vi "Waveform-Processing-Custom-Device.Async.vi"(10 "Parameters":variant, 11 "Process":refnum<class "Process.lvclass">) -> ()   [LabVIEW 2017, in "Waveform-Processing-Custom-Device Engine.lvlib"]
uses:
  Waveform-Processing-Custom-Device Engine.lvlib
  <vilib>/NI/NIVS Inline Async API/_VS Inline Async API/Process/Process.lvclass
  Shared/CompiledSettings.ctl
  <vilib>/NI Veristand/Custom Device API/Block Data Reference.ctl
  <vilib>/NI Veristand/Custom Device API/Data Reference.ctl
  <vilib>/NI Veristand/Custom Device API/Waveform Data Reference.ctl
  <vilib>/NI/NIVS Inline Async API/_VS Inline Async API/Process/Process.lvclass/Process.ctl
  <vilib>/NI/NIVS Inline Async API/_VS Inline Async API/Process/Data Member Access/Read Data Access.vi
  <vilib>/NI/NIVS Inline Async API/_VS Inline Async API/Error Handling Process/SubVIs/Error.ConvertArray.vi
  <vilib>/NI/NIVS Inline Async API/_Data Access Engine/Data Access Engine/Data Access Engine.lvclass
  Shared/Running Average/Running Average.lvlib
  Shared/Single Point/SinglePoint.lvlib
  <vilib>/NI Veristand/Custom Device API/Custom Device API.lvlib
  Shared/Waveform-Processing-Custom-Device Shared.lvlib
  Shared/Min Single Point/Min_SP.lvlib
  Shared/Max Single Point/Max_SP.lvlib
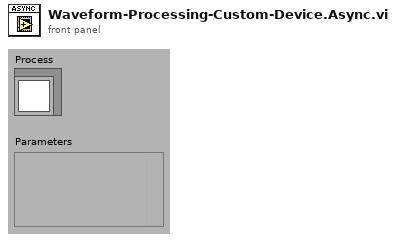
[diagram p1: front panel]
types:
  T1 = typedef "Waveform-Processing-Custom-Device Shared.lvlib/CompiledSettings.ctl" = cluster{"Name":string, "Buffer Length (samples)":u32, "Enable Array":bool[], "Parameter Block Data Refs":T2[], "Source Wfm Data Refs":T4[], "Result Wfm Data Refs":T4[], "Result Ch Data Refs":T3[], "Task Rate (Hz)":dbl}
  T2 = typedef "Custom Device API.lvlib/Block Data Reference.ctl" = cluster{"Data Reference":T3, "Offset":u64, "Length":u64}
  T3 = typedef "Custom Device API.lvlib/Data Reference.ctl" = i32
  T4 = typedef "Custom Device API.lvlib/Waveform Data Reference.ctl" = i32
  T5 = typedef "Waveform-Processing-Custom-Device Engine.lvlib/AsyncStateVariables.ctl" = cluster{"Source Wfm Session Refs":refnum<class "Single Waveform Read (DBL).lvclass">[], "Result Wfm Session Refs":refnum<class "Single Waveform Write (DBL).lvclass">[], "Result Wfm Data":dbl[][], "Source Wfm Data Refs":T4[], "Result Wfm Data Refs":T4[], "Global Buffer Length (samples)":dbl, "Parameter Array":dbl[], "Tag Results":dbl[], "Enable Array":bool[], "Task Rate":dbl, "Data FIFO Refs":T6}
  T6 = typedef "Waveform-Processing-Custom-Device Engine.lvlib/New Async FIFOs.ctl" = cluster{"Single Point Result":T7, "Running Average Result":T7, "Min Single Point Result":T7, "Max Single Point Result ":T7}
  T7 = typedef "Data Access Engine.lvlib/Data Access Engine.lvclass/Write.DVR.ctl" = refnum<data-value>
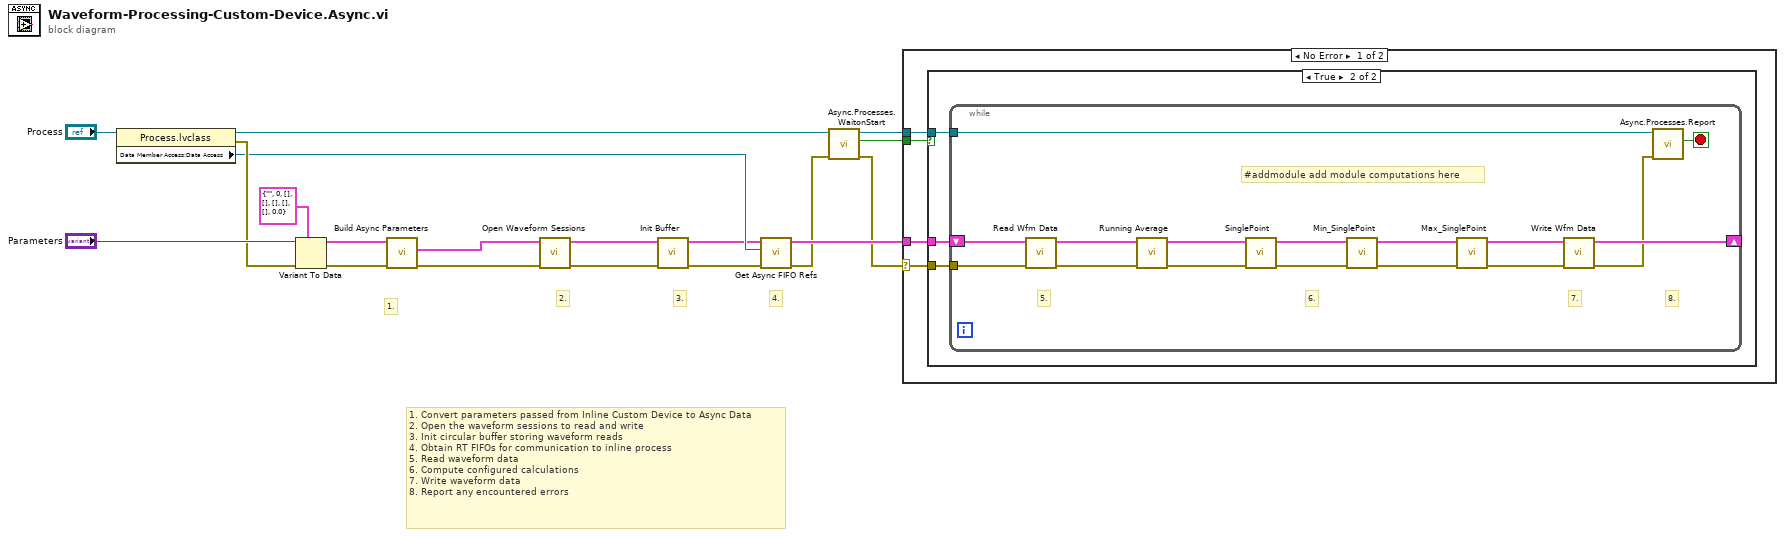
[diagram p0: block diagram]
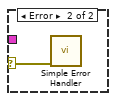
[diagram p3: hidden frame]
diagram:
  # "4."
  # "3."
  # "2."
  # "1."
  # "1. Convert parameters passed from Inline Custom Device to Async Data\n2. Open the waveform sessions to read and write\n3. Init circular buffer storing waveform reads\n4. Obtain RT FIFOs for communication to inline process\n5. Read waveform data\n6. Compute configured calculations\n7. Write waveform data\n8. Report any encountered errors"
  n1 = property class="Process.lvclass"(reference="Process") -> (reference out=w16:refnum<class "Process.lvclass">, error out=w14:errorcluster, "Data Member Access:Data Access"=w12:refnum<class "Data Access Engine.lvclass">)  [unwired: 1 in]
  n2 = Variant To Data(error in=w14, type=T1 {"Name"="", "Buffer Length (samples)"=0, "Enable Array"=[], "Parameter Block Data Refs"=[], "Source Wfm Data Refs"=[], "Result Wfm Data Refs"=[], "Result Ch Data Refs"=[], "Task Rate (Hz)"=0.0} ("CompiledSettings"), Variant="Parameters") -> (data=w8:T1, error out=w5:errorcluster)
  n3 = call "Build Async Parameters.vi"("Error in"=w5, "CompiledSettings In"=w8) -> ("Error out"=w4:errorcluster, "Async State Vars"=w9:T5)  [unwired: 7 in, 1 out]
  n4 = call "Open Waveform Sessions.vi"("error in"=w4, "Async State Vars"=w9) -> ("error out"=w3:errorcluster, "Async State Vars out"=w13:T5)  [unwired: 8 in]
  n5 = call "Init Buffer.vi"("Error in"=w3, "Async State Vars"=w13) -> ("Error out"=w2:errorcluster, "Async State Vars out"=w11:T5)  [unwired: 8 in]
  n6 = call "Get Async FIFO Refs.vi"("error in"=w2, "Data Access API In"=w12, "Async State Vars In"=w11) -> ("error out"=w1:errorcluster, "Async State Vars Out"=w10:T5)  [unwired: 6 in, 1 out]
  n7 = call <vilib>:"Async.Processes.WaitonStart.vi"("error in (no error)"=w1, "Process"=w16) -> ("error out"=w7:errorcluster, "Execute"=w19:bool, "Process out"=w18:refnum<class "Process.lvclass">)  [unwired: 7 in]
  n8 = case shown="No Error" w7 {
    selector: w7 -> [w21 w43]
    tunnel: w19 -> [w23 _]
    tunnel: w18 -> [w22 _]
    tunnel: w10 -> [w20 _]
    frame No Error {
      n9 = case shown="True" w23 {
        tunnel: w21 -> [_ w25]
        tunnel: w22 -> [_ w26]
        tunnel: w20 -> [_ w24]
        frame False {
        }
        frame True {
          n10 = while {
            tunnel: w25 -> [w35]
            tunnel: w26 -> [w42]
            shift-right: [w38] -> _
            shift-left: w24 -> [w40]
            stop <- w41 stop-if-true
            # "#addmodule add module computations here"
            # "8."
            # "7."
            # "6."
            # "5."
            n11 = call "Read Wfm Data.vi"("error in"=w35, "Async State Vars in"=w40) -> ("error out"=w29:errorcluster, "Async State Vars out"=w39:T5)  [unwired: 7 in, 1 out]
            n12 = call "Running Average.vi"("Error In"=w29, "Async State Vars In"=w39) -> ("Error Out"=w36:errorcluster, "Async State Vars out"=w37:T5)  [unwired: 8 in]
            n13 = call "SinglePoint.vi"("Error In"=w36, "Async State Vars In"=w37) -> ("Error Out"=w31:errorcluster, "Async State Vars out"=w33:T5)  [unwired: 8 in]
            n14 = call "Min_SinglePoint.vi"("Error In"=w31, "Async State Vars In"=w33) -> ("Error Out"=w28:errorcluster, "Async State Vars out"=w34:T5)  [unwired: 8 in]
            n15 = call "Max_SinglePoint.vi"("Error In"=w28, "Async State Vars In"=w34) -> ("Error Out"=w30:errorcluster, "Async State Vars out"=w32:T5)  [unwired: 8 in]
            n16 = call "Write Wfm Data.vi"("error in"=w30, "Async State Vars in"=w32) -> ("error out"=w27:errorcluster, "Async State Vars out"=w38:T5)  [unwired: 7 in, 1 out]
            n17 = call <vilib>:"Async.Processes.Report.vi"("Error"=w27, "Process in"=w42) -> ("Stop"=w41:bool)  [unwired: 8 in, 1 out]
          }
        }
      }
    }
    frame Error {
      n18 = call <vilib>:"Simple Error Handler.vi"("error in (no error)"=w43) -> ()  [unwired: 4 in, 5 out]
    }
  }
